vi "Mono SubVI Test Structure - Copy.vi"() -> ()   [LabVIEW 2015]
uses:
  K:/OSSIP/Optical Test Setup/System Qualification/LabVIEW Development/Cornerstone.dll
panel:
  out "Wavelength Set?":bool=TRUE
  in  "Wavelength":dbl format="%#_13g"
  out ".NET Refnum":refnum<k24>
  out "error out":errorcluster
  in  "error in (no error)":errorcluster
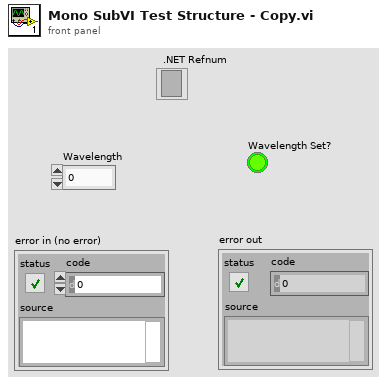
[diagram p1: front panel]
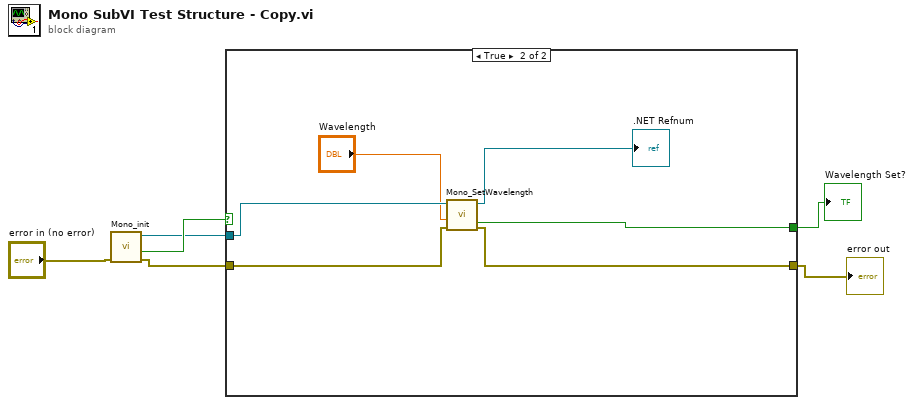
[diagram p0: block diagram]
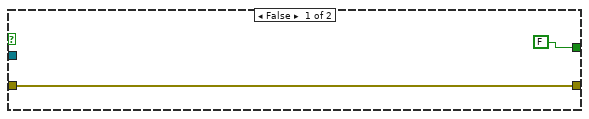
[diagram p2: hidden frame]
diagram:
  n1 = call "Mono_init.vi"("error in (no error)"="error in (no error)") -> ("error out"=w6:errorcluster, "Mono Connected?"=w5:bool, "CmdLib"=w2:refnum<k24>)  [unwired: 8 in]
  n2 = case shown="True" w5 {
    tunnel: w6 -> [w8 w12]
    tunnel: [w8 w11] -> w3
    tunnel: w2 -> [_ w14]
    tunnel: [FALSE w9] -> w1
    frame False {
    }
    frame True {
      n3 = call "Mono_SetWavelength.vi"("error in (no error) 2"=w12, "Wavelength"="Wavelength", "CmdLib In"=w14) -> ("error out 2"=w11:errorcluster, "Wavelength Set"=w9:bool, "CmdLib Out"=→".NET Refnum":refnum<k24>)  [unwired: 6 in]
    }
  }
  "error out" <- w3
  "Wavelength Set?" <- w1
